vi "SC10_get_shutter_state.vi"() -> ()   [LabVIEW 2010]
panel:
  out "substring":string
  in  "VISA resource name":refnum<visa-resource-name>
  out "VISA resource name out":refnum<visa-resource-name>
  out "read buffer":string
  out "return count 2":u32
  out "return count":u32
  out "error out":errorcluster
  in  "error in (no error)":errorcluster
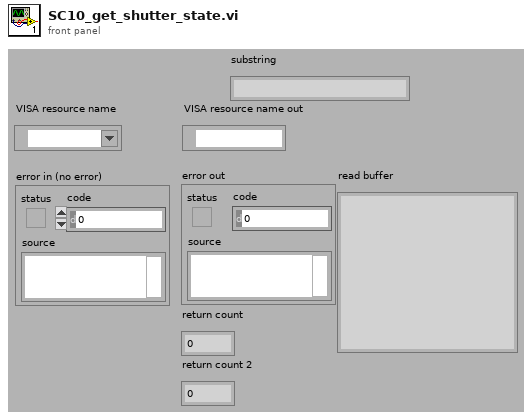
[diagram p1: front panel]
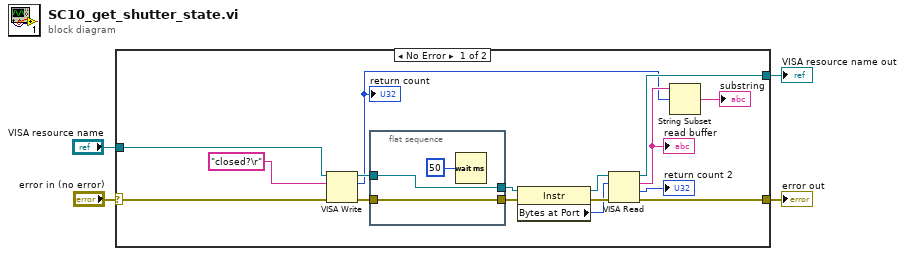
[diagram p0: block diagram]
diagram:
  n1 = case shown="No Error" "error in (no error)" {
    selector: "error in (no error)" -> [w18 w24]
    tunnel: [w17 w24] -> w3
    tunnel: [w15 w25] -> w2
    tunnel: "VISA resource name" -> [w14 w25]
    frame No Error {
      n2 = VISA Write(VISA resource name=w14, write buffer="closed?\r", error in (no error)=w18) -> (VISA resource name out=w20:refnum<visa-resource-name>, return count=w11:u32, error out=w19:errorcluster)
      "return count" <- w11
      n3 = flat-sequence {
        tunnel: w20 -> [w22]
        tunnel: [w22] -> w8
        tunnel: w19 -> [w21]
        tunnel: [w21] -> w7
        frame #0 {
          n4 = Wait (ms)(milliseconds to wait=u32 50) -> ()  [unwired: 1 out]
        }
      }
      n5 = property class="Instr"(reference=w8, error in=w7) -> (reference out=w9:refnum<visa-resource-name>, error out=w10:errorcluster, "Bytes at Port"=w6:u32)
      n6 = VISA Read(VISA resource name=w9, byte count=w6, error in (no error)=w10) -> (VISA resource name out=w15:refnum<visa-resource-name>, read buffer=w13:string, return count=→"return count 2":u32, error out=w17:errorcluster)
      "read buffer" <- w13
      n7 = String Subset(string=w13, offset (0)=w11) -> (substring=→"substring":string)  [unwired: 1 in]
    }
    frame Error {
    }
  }
  "error out" <- w3
  "VISA resource name out" <- w2
